vi "PartialClusters2.vi"(5 "ClusterInput":cluster{"Array":dbl[][]}={"Array"=[[1.0, 2.0, 3.0, 4.0, 5.0, 6.0], [1.0, 0.0, 0.0, 0.0, 0.0, 0.0], [2.0, 0.0, 0.0, 0.0, 0.0, 0.0], [3.0, 0.0, 0.0, 0.0, 0.0, 0.0], [4.0, 0.0, 0.0, 0.0, 0.0, 0.0], [6.0, 0.0, 0.0, 0.0, 0.0, 0.0]]}) -> (0 "x = y?":bool=TRUE, 1 "sum":dbl=36.0, 2 "MySum":dbl=36.0)   [LabVIEW 2012]
panel:
  in  "Init Value":dbl
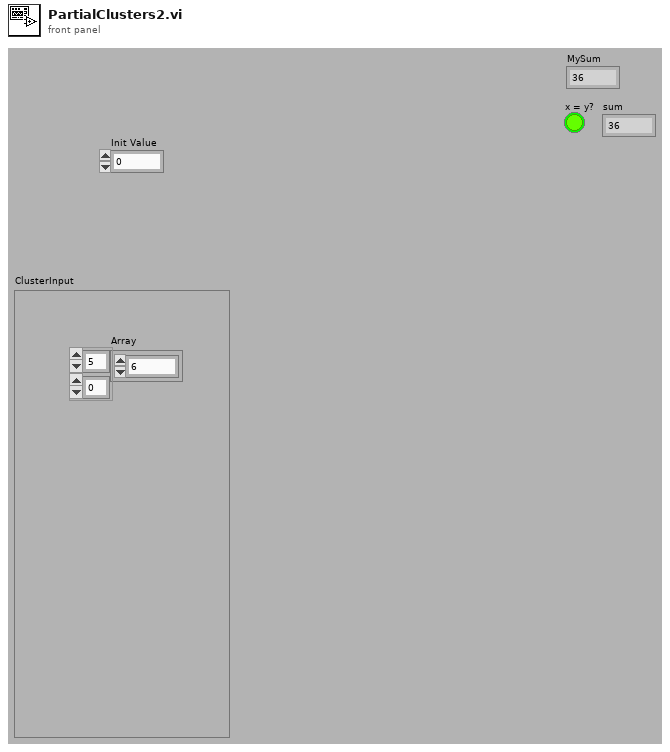
[diagram p1: front panel]
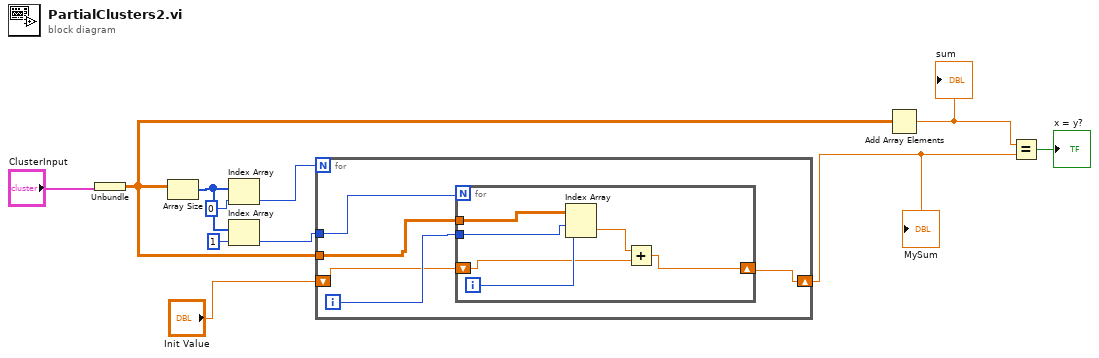
[diagram p0: block diagram]
diagram:
  n1 = Unbundle("ClusterInput") -> ("Array"=w5:dbl[][])
  n2 = Array Size(array=w5) -> (size(s)=w9:i32[])
  n3 = Index Array(array=w9, index=0) -> (element=w7:i32)
  n4 = Index Array(array=w9, index=1) -> (element=w6:i32)
  n5 = for {
    N: w7 -> [_]
    tunnel: w6 -> [w16]
    tunnel: w5 -> [w14]
    shift-right: [w12] -> w2
    shift-left: "Init Value" -> [w13]
    i -> [w15]
    n6 = for {
      N: w16 -> [_]
      tunnel: w15 -> [w21]
      tunnel: w14 -> [w22]
      shift-right: [w17] -> w12
      shift-left: w13 -> [w19]
      i -> [w20]
      n7 = Index Array(array=w22, index (row)=w21, index (col)=w20) -> (element=w18:dbl)
      n8 = Add(x=w18, y=w19) -> (x+y=w17:dbl)
    }
  }
  "MySum" <- w2
  n9 = Add Array Elements(numeric array=w5) -> (sum=w3:dbl)
  "sum" <- w3
  n10 = Equal?(x=w3, y=w2) -> (x = y?=→"x = y?":bool)
